vi "Get Slide Text.vi"(8 "error in (no error)":errorcluster, 11 "Parse Presentation in":refnum<class "Parse Presentation.lvclass">) -> (0 "error out":errorcluster, 3 "Parse Presentation out":refnum<class "Parse Presentation.lvclass">)   [LabVIEW 2015, in "Parse Presentation.lvclass"]
uses:
  Parse Presentation.lvclass
  Parse Presentation.lvclass/Parse Presentation.ctl
  D:/Metis Automation/ppt-parsing/LabVIEW/DLL/ParsePpt.dll
  DLL/ParsePpt.dll
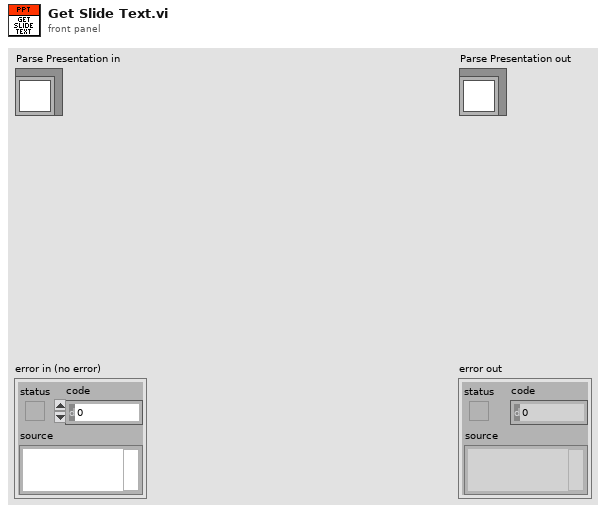
[diagram p1: front panel]
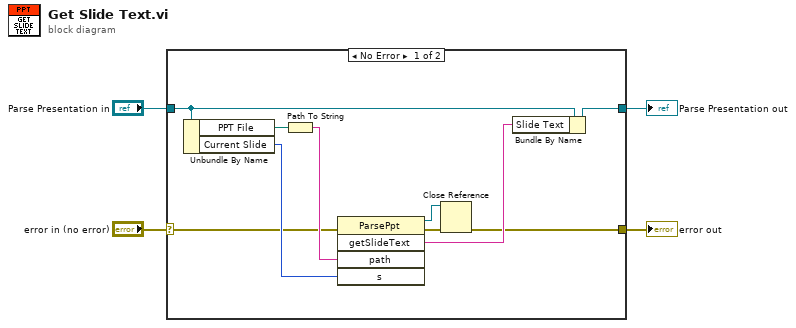
[diagram p0: block diagram]
diagram:
  n1 = case shown="No Error" "error in (no error)" {
    selector: "error in (no error)" -> [w10 w16]
    tunnel: [w6 w16] -> w3
    tunnel: [w8 w15] -> w1
    tunnel: "Parse Presentation in" -> [w14 w15]
    frame No Error {
      n2 = Unbundle By Name(w14) -> ("PPT File"=w13:path, "Current Slide"=w11:i32)
      n3 = Path To String(path=w13) -> (string=w12:string)
      n4 = invoke class="ParsePpt" method="getSlideText"(error in=w10, "path"=w12, "s"=w11) -> (reference out=w5:refnum<k24>, error out=w9:errorcluster, "getSlideText"=w7:string)  [unwired: 2 in, 2 out]
      n5 = Close Reference(reference=w5, error in (no error)=w9) -> (error out=w6:errorcluster)
      n6 = Bundle By Name(cluster=w14, "Slide Text"=w7) -> (w8:refnum<class "Parse Presentation.lvclass">)
    }
    frame Error {
    }
  }
  "error out" <- w3
  "Parse Presentation out" <- w1
